vi "Delete Flat BOM Rows.vi"(8 "error in (no error)":errorcluster, 11 "Data":T1) -> (0 "error out":errorcluster, 3 "OK":bool)   [LabVIEW 2018]
uses:
  TypeDef/Main - Handle Heirarchy Drag&Drop - Data.ctl
  <vilib>/httpClient/LabVIEWHTTPClient.lvlib
panel:
  out "Bodies":string[](array[string])
  out "Headers":string[](array[string])
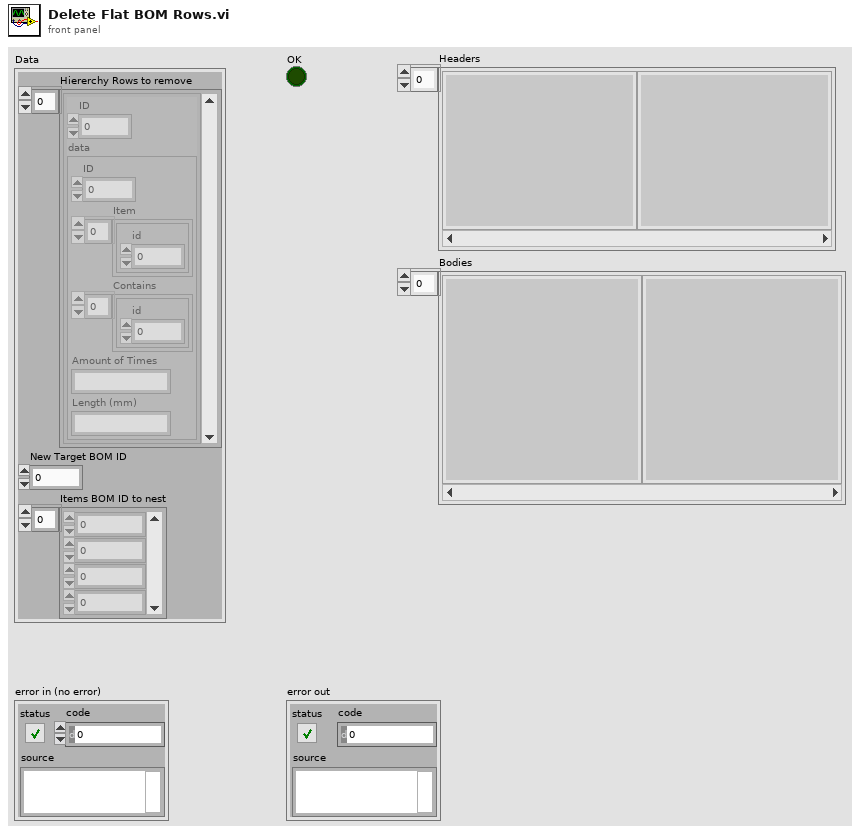
[diagram p1: front panel]
types:
  T1 = typedef "Main - Handle Heirarchy Drag&Drop - Data.ctl" = cluster{"Hiererchy Rows to remove":cluster{"ID":i32, "data":cluster{"ID":i32, "Item":cluster{"id":i32}[], "Contains":cluster{"id":i32}[], "Amount of Times":string, "Length (mm)":string}}[], "New Target BOM ID":i32, "Items BOM ID to nest":i32[]}
  T2 = typedef "LabVIEWHTTPClient.lvlib/ClientHandle.ctl" = refnum<k1>
  T3 = cluster{"ID":i32, "data":cluster{"ID":i32, "Item":cluster{"id":i32}[], "Contains":cluster{"id":i32}[], "Amount of Times":string, "Length (mm)":string}}[]
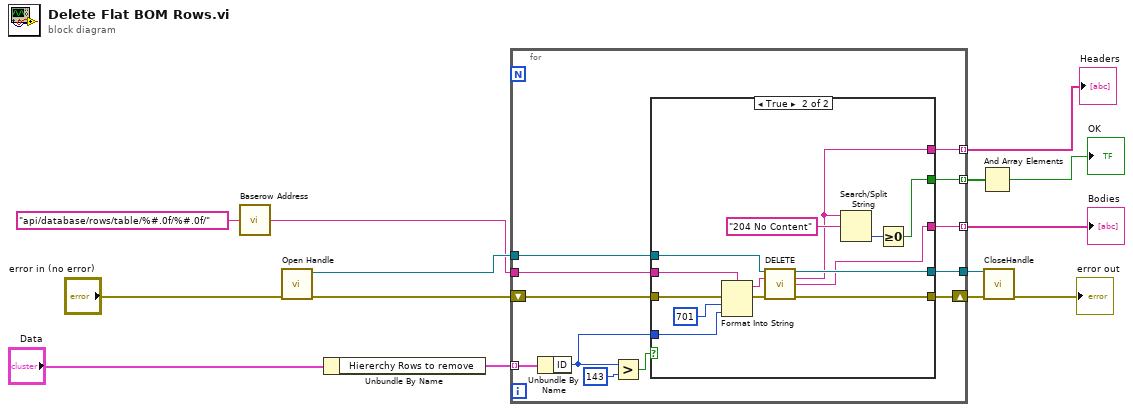
[diagram p0: block diagram]
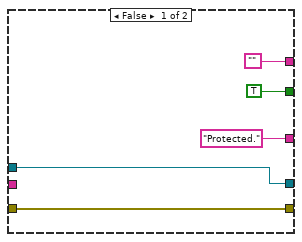
[diagram p2: hidden frame]
diagram:
  n1 = call "Baserow Address.vi"("Path"="api/database/rows/table/%#.0f/%#.0f/" ("url")) -> ("URL + Path"=w2:string)
  n2 = call "Open Handle.vi"("error in (no error)"="error in (no error)") -> ("error out"=w12:errorcluster, "Refnum out"=w10:T2)  [unwired: 9 in]
  n3 = Unbundle By Name("Data") -> ("Hiererchy Rows to remove"=w11:T3)
  n4 = for {
    tunnel: w2 -> [w25]
    shift-right: [w26] -> w9
    shift-left: w12 -> [w24]
    tunnel: w11 -> [w18] mode=indexing
    tunnel: w10 -> [w23]
    tunnel: [w22] -> w7
    tunnel: [w20] -> w6 mode=indexing
    tunnel: [w21] -> w5 mode=indexing
    tunnel: [w19] -> w4 mode=indexing
    n5 = Unbundle By Name(w18) -> ("ID"=w16:i32)
    n6 = Greater?(x=w16, y=u32 143 ("input 1")) -> (0:w15:bool)
    n7 = case shown="True" w15 {
      tunnel: [w30 w45] -> w26
      tunnel: w25 -> [_ w44]
      tunnel: w24 -> [w30 w42]
      tunnel: w23 -> [w28 w39]
      tunnel: [w28 w38] -> w22
      tunnel: ["Protected." ("body") w37] -> w21
      tunnel: ["" w34] -> w20
      tunnel: [TRUE w33] -> w19
      tunnel: w16 -> [_ w32]
      frame False {
      }
      frame True {
        n8 = Format Into String(format string=w44, error in=w42, u32 701 ("input 1"), w32) -> (resulting string=w40:string, error out=w41:errorcluster)  [unwired: 1 in]
        n9 = call <vilib>:"DELETE.vi"("client handle"=w39, "url"=w40, "error in (no error)"=w41) -> ("client handle out"=w38:T2, "headers"=w34:string, "body"=w37:string, "error out"=w45:errorcluster)  [unwired: 9 in]
        n10 = Search/Split String(string=w34, search string/char (-)="204 No Content") -> (offset of match=w35:i32)  [unwired: 1 in, 2 out]
        n11 = Greater Or Equal To 0?(x=w35) -> (x >= 0?=w33:bool)
      }
    }
  }
  "Bodies" <- w5
  "Headers" <- w6
  n12 = And Array Elements(Boolean array=w4) -> (logical AND=→"OK":bool)
  n13 = call <vilib>:"CloseHandle.vi"("client handle"=w7, "error in (no error)"=w9) -> ("error out"=→"error out":errorcluster)  [unwired: 13 in]
